vi "arduino_thermal.vi"() -> ()   [LabVIEW 2013]
uses:
  <vilib>/LabVIEW Interface for Arduino/LabVIEW Interface for Arduino.lvlib
panel:
  out "Thermometer":dbl(slide) scale=0.0..100.0
  in  "stop":bool
  in  "Paired Resistance (10K Ohms)":dbl=10000.0
  in  "Thermistor AI Pin (0)":u8
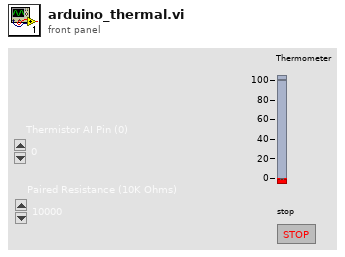
[diagram p1: front panel]
types:
  T1 = typedef "LabVIEW Interface for Arduino.lvlib/Arduino Resource.ctl" = cluster{"VISA resource":refnum<visa-resource-name>, "Board Type":T2, "Connection Type":enum8{"USB / Serial"}, "Bytes Per Packet (15)":u8}
  T2 = typedef "LabVIEW Interface for Arduino.lvlib/Board Type.ctl" = enum16{"Uno", "Dimuelanove w/Atmega 328", "Mega 2560"}
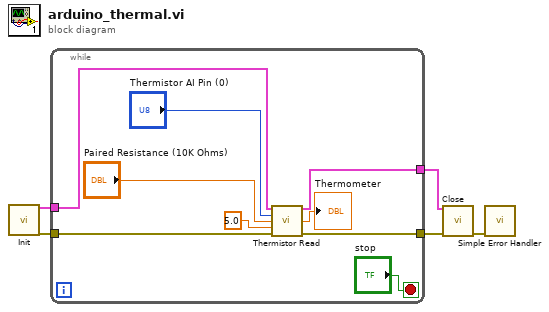
[diagram p0: block diagram]
diagram:
  n1 = call <vilib>:"Init.vi"() -> ("Arduino Resource"=w2:T1, "error out"=w5:errorcluster)  [unwired: 18 in]
  n2 = while {
    tunnel: w5 -> [w11]
    tunnel: [w10] -> w4
    tunnel: w2 -> [w9]
    tunnel: [w8] -> w1
    stop <- "stop" stop-if-true
    n3 = call <vilib>:"Thermistor Read.vi"("Arduino Resource"=w9, "Thermistor AI Pin (0)"="Thermistor AI Pin (0)", "Paired Resistance (10K Ohms)"="Paired Resistance (10K Ohms)", "Vcc (5 v)"=5.0, "error in"=w11) -> ("Arduino Resource"=w8:T1, "Temperature"=→"Thermometer":dbl, "error out"=w10:errorcluster)  [unwired: 8 in]
  }
  n4 = call <vilib>:"Close.vi"("Arduino Resource"=w1, "error in"=w4) -> ("error out"=w3:errorcluster)  [unwired: 13 in]
  n5 = call <vilib>:"Simple Error Handler.vi"("error in (no error)"=w3) -> ()  [unwired: 4 in, 5 out]
